vi "GPS_file_viewer.vi"() -> ()   [LabVIEW 2009]
uses:
  <vilib>/Utility/file.llb/Read From Spreadsheet File (DBL).vi
  <vilib>/Platform/NI_3dgraph.lvlib
panel:
  out "XY Graph":cluster{"Y":dbl[], "Y":dbl[]}[](graph)
  out "northing":dbl[](graph)
  out "easting":dbl[](graph)
  out "Altitude":dbl[](graph)
  in  "3D Curve - Lorenz Attractor":refnum<k7>(container)
  out "altitude":dbl[](array[numeric])
  out "northing":dbl[](array[numeric])
  out "easting":dbl[](array[numeric])
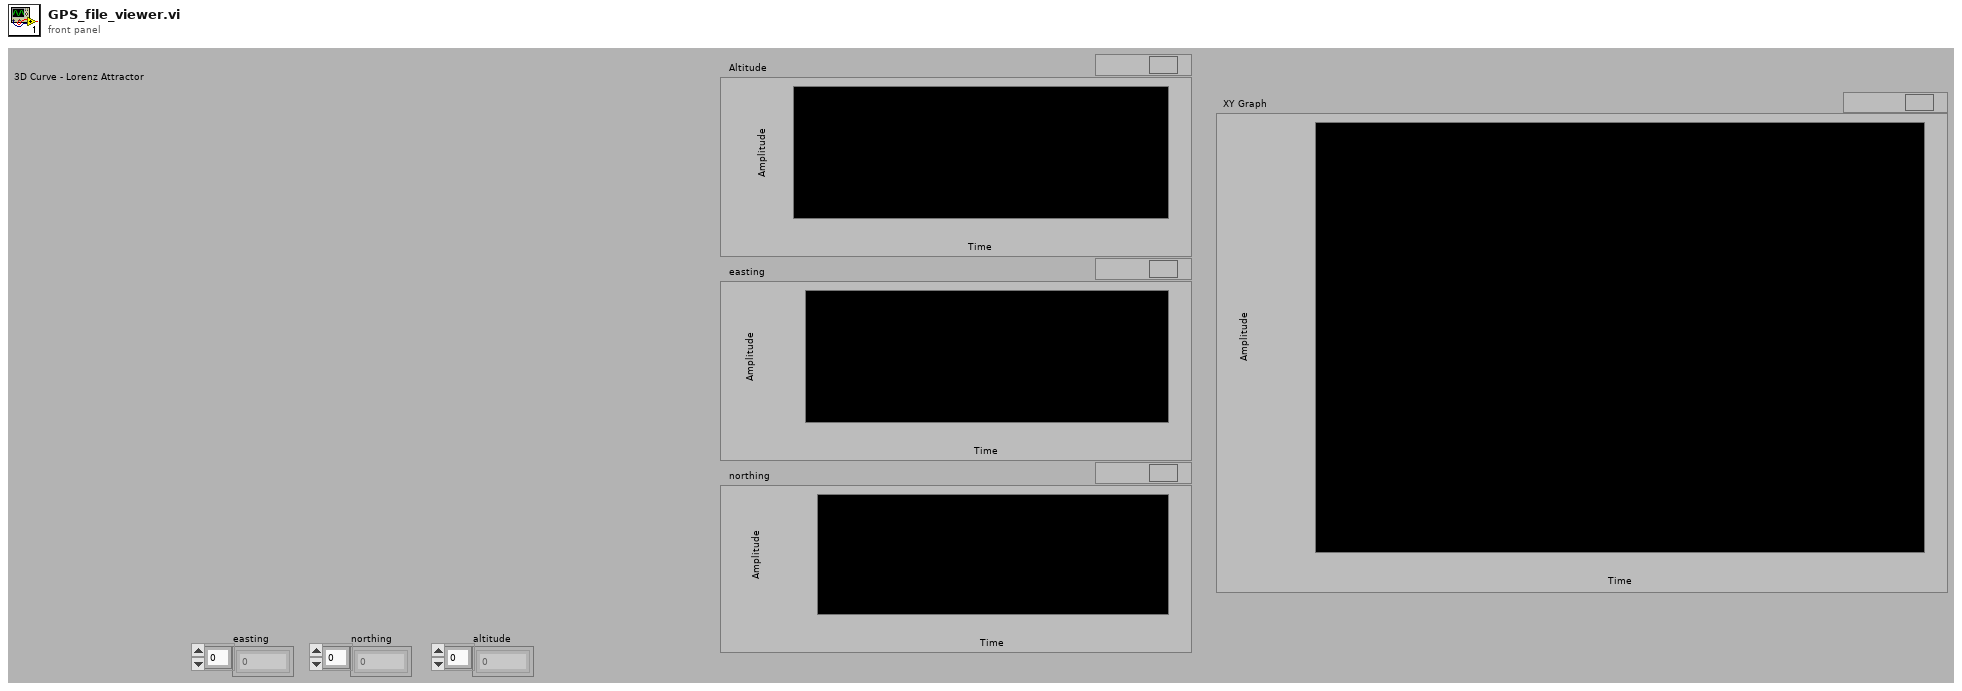
[diagram p1: front panel]
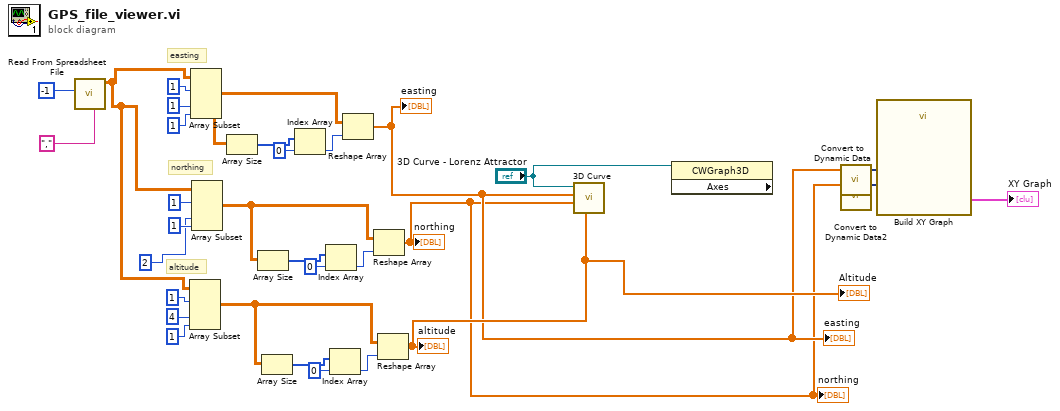
[diagram p0: block diagram]
diagram:
  # "altitude"
  # "northing"
  # "easting"
  n1 = call-poly <vilib>:"Read From Spreadsheet File.vi"("delimiter (\\t)"="," ("delimiter (\\t)"), "number of rows (all:-1)"=-1) -> ("all rows"=w20:dbl[][])  [unwired: 5 in, 4 out]
  n2 = Array Subset(array=w20, index (row)=1 ("index"), index (col)=4 ("index"), length (col)=1 ("length")) -> (w8:dbl[][])  [unwired: 1 in]
  n3 = Array Subset(array=w20, index (row)=1 ("index"), index (col)=1 ("index"), length (col)=1 ("length")) -> (w16:dbl[][])  [unwired: 1 in]
  n4 = Array Subset(array=w20, index (row)=1 ("index"), index (col)=2 ("index"), length (col)=1 ("length")) -> (w9:dbl[][])  [unwired: 1 in]
  n5 = Array Size(array=w16) -> (size(s)=w19:i32[])
  n6 = Array Size(array=w9) -> (size(s)=w13:i32[])
  n7 = Array Size(array=w8) -> (size(s)=w12:i32[])
  n8 = Index Array(array=w19, index=0) -> (element=w17:i32)
  n9 = Index Array(array=w13, index=0) -> (element=w15:i32)
  n10 = Index Array(array=w12, index=0) -> (element=w10:i32)
  n11 = Reshape Array(w16, w17) -> (w4:dbl[])
  "easting" <- w4
  "easting" <- w4
  n12 = Reshape Array(w9, w15) -> (w2:dbl[])
  "northing" <- w2
  "northing" <- w2
  n13 = Reshape Array(w8, w10) -> (w6:dbl[])
  "altitude" <- w6
  "Altitude" <- w6
  n14 = call <vilib>:"3D Curve.vi"("z vector"=w6, "y vector"=w2, "x vector"=w4, "3D graph"="3D Curve - Lorenz Attractor") -> ()  [unwired: 6 in, 2 out]
  n15 = property class="CWGraph3D" props=["Axes"](reference="3D Curve - Lorenz Attractor") -> ()  [unwired: 1 in, 3 out]
  n16 = call "Convert to Dynamic Data"("Array"=w4) -> ("Dynamic Data Type"=w3:dynamicdata)  [unwired: 3 in]
  n17 = call "Convert to Dynamic Data2"("Array"=w2) -> ("Dynamic Data Type"=w1:dynamicdata)  [unwired: 3 in]
  n18 = call "Build XY Graph"("Y Input"=w1, "X Input"=w3) -> ("XY Graph"=→"XY Graph":cluster{"Y":dbl[], "Y":dbl[]}[])  [unwired: 8 in, 1 out]
